vi "Check Reserve Levels.vi"(8 "error in (no error)":errorcluster, 11 "Data":T1) -> (0 "error out":errorcluster, 3 "Reserves Low?":bool)   [LabVIEW 2026]
uses:
  controls/Data.ctl
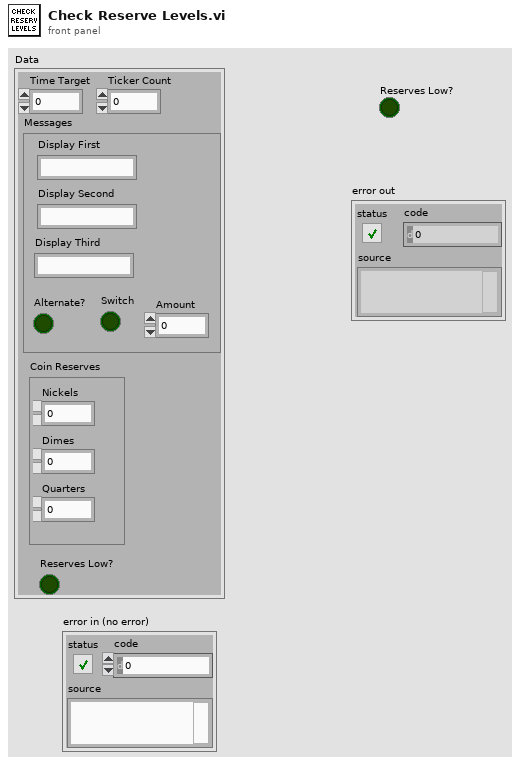
[diagram p1: front panel]
types:
  T1 = typedef "Data.ctl" = cluster{"Time Target":dbl, "Messages":cluster{"Display First":string, "Display Second":string, "Alternate?":bool, "Switch":bool, "Display Third":string, "Amount":i32}, "Ticker Count":dbl, "Coin Reserves":cluster{"Nickels":i32, "Dimes":i32, "Quarters":i32}, "Reserves Low?":bool}
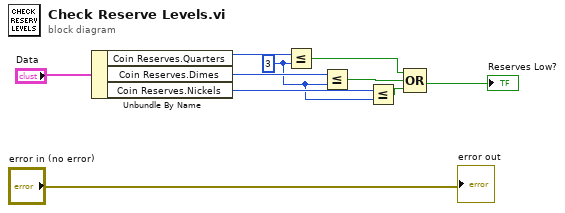
[diagram p0: block diagram]
diagram:
  w3 = 3 ("y")
  n1 = Unbundle By Name("Data") -> ("Coin Reserves.Quarters"=w7:i32, "Coin Reserves.Dimes"=w8:i32, "Coin Reserves.Nickels"=w9:i32)
  n2 = Less Or Equal?(x=w7, y=w3) -> (x <= y?=w4:bool)
  n3 = Less Or Equal?(x=w8, y=w3) -> (x <= y?=w5:bool)
  n4 = Less Or Equal?(x=w9, y=w3) -> (x <= y?=w6:bool)
  n5 = Compound Arithmetic op=OR(w4, w5, w6) -> (→"Reserves Low?":bool)
  "error out" <- "error in (no error)"
